vi "setLabelProperties.vi"(6 "visible":bool, 8 "error in (no error)":errorcluster, 10 "label":string, 11 "Wire in":refnum<class "Wire.lvclass">) -> (0 "error out":errorcluster, 3 "Wire in":refnum<class "Wire.lvclass">)   [LabVIEW 2023, in "TLC_Scripto.lvlib" / "Wire.lvclass"]
uses:
  Wire.lvclass
  Wire.lvclass/Wire.ctl
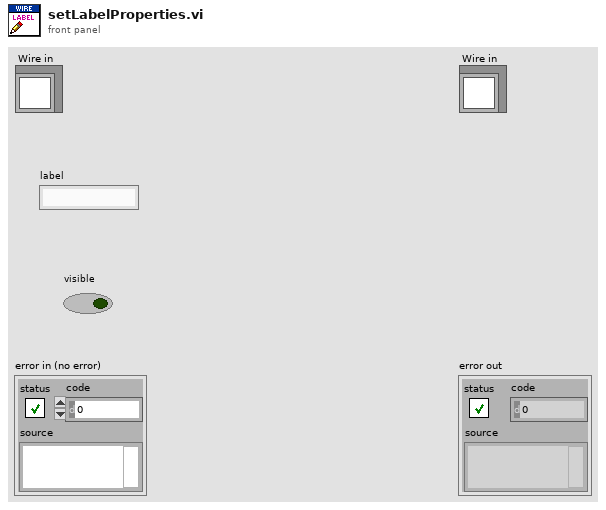
[diagram p1: front panel]
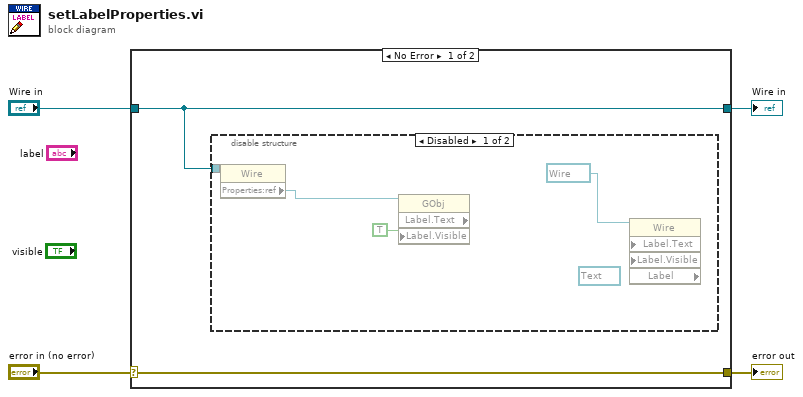
[diagram p0: block diagram]
diagram:
  n1 = case shown="No Error" "error in (no error)" {
    selector: "error in (no error)" -> [w6 w13]
    tunnel: [w6 w13] -> w3
    tunnel: [w5 w12] -> w1
    tunnel: "Wire in" -> [w5 w12]
    frame No Error {
      n2 = disable-structure shown="Disabled" {
        disable-tunnel: w5 -> [w9 _]
        frame Disabled {
          (unwired) refnum<vi> refnum ("Label")
          n3 = property class="Wire"(reference=w9) -> ("Properties:ref"=w8:refnum<vi>)  [unwired: 1 in, 2 out]
          n4 = property class="GObj"(reference=w8, "Label.Visible"=TRUE) -> ("Label.Text"=w11)  [unwired: 1 in, 2 out]
          n5 = property class="Wire" props=["Label", "Text", "Label", "Visible", "Label"](reference=refnum<vi> refnum ("ref")) -> ()  [unwired: 3 in, 3 out]
        }
        frame Enabled {
        }
      }
    }
    frame Error {
    }
  }
  "error out" <- w3
  "Wire in" <- w1
